vi "Pololu.Mgr - Connect.vi"(8 "error in (no error)":errorcluster, 9 "PID":string, 10 "VID":string, 11 "PololuCtrl in":refnum<class "PololuCtrl.lvclass">) -> (0 "error out":errorcluster, 2 "Com Port":refnum<visa-resource-name>, 3 "PololuCtrl out":refnum<class "PololuCtrl.lvclass">)   [LabVIEW 2018, in "PololuCtrl.lvclass"]
uses:
  PololuCtrl.lvclass
  Utils/Errors/Error.Error Code List.ctl
  PololuCtrl.lvclass/PololuCtrl.ctl
  Serial Port/Class/SerialPort.lvclass
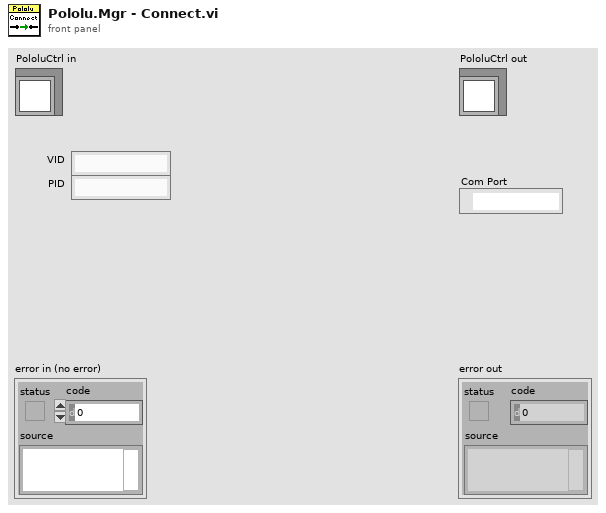
[diagram p1: front panel]
types:
  T1 = typedef "Error.Error Code List.ctl" = i32
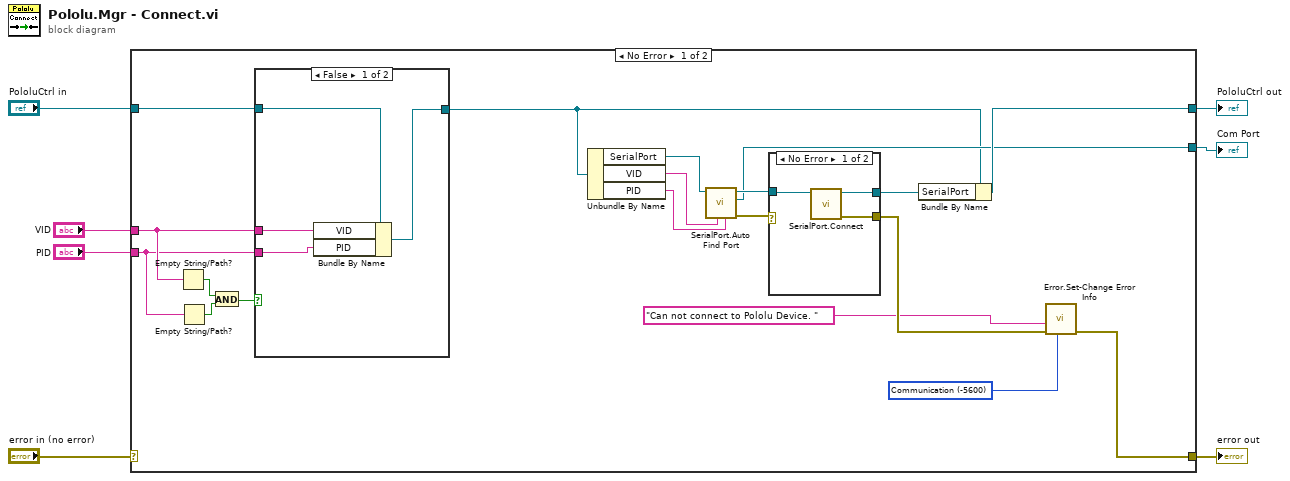
[diagram p0: block diagram]
diagram:
  n1 = case shown="No Error" "error in (no error)" {
    selector: "error in (no error)" -> [_ w38]
    tunnel: [w16 w38] -> w6
    tunnel: [w26 w37] -> w4
    tunnel: "PololuCtrl in" -> [w11 w37]
    tunnel: [w15 _] -> w3
    tunnel: "VID" -> [w9 _]
    tunnel: "PID" -> [w8 _]
    frame No Error {
      w18 = T1 -5600 items=["No Error"=0, "Abort"=-2, "Misc"=-5000, "Fixture Error"=-5100, "File IO - General"=-5200, "FIle IO - Config Error"=-5201, "Instrument - General"=-5300, "Instrument - Serial Com"=-5301, "Instrument - Camera"=-5302, "Instrument - PS"=-5303, "Instrument - Oscilloscope"=-5304, "Instrument - Function Gen"=-5305, "Instrument - Load"=-5306, "Instrument - Meter"=-5307, "Instrument - Power Control"=-5308, "Instrument - Motion"=-5309, "Instrument - RF"=-5310, "System Exe"=-5400, "Image Processing"=-5500, "Communication"=-5600, "Script - Syntax Error"=-6000, "Script - Invalid Name or Param"=-6100, "Script - Timeout"=-6200, "Invalid Data"=-6300, "FW Update Error"=-6500] ("Std Code")
      n2 = Empty String/Path?(string/path=w9) -> (empty?=w13:bool)
      n3 = Empty String/Path?(string/path=w8) -> (empty?=w14:bool)
      n4 = And(x=w13, y=w14) -> (x .and. y?=w12:bool)
      n5 = case shown="False" w12 {
        tunnel: w11 -> [w30 w31]
        tunnel: [w27 w31] -> w10
        tunnel: w9 -> [w29 _]
        tunnel: w8 -> [w28 _]
        frame False {
          n6 = Bundle By Name(cluster=w30, "VID"=w29, "PID"=w28) -> (w27:refnum<class "PololuCtrl.lvclass">)
        }
        frame True {
        }
      }
      n7 = Unbundle By Name(w10) -> ("SerialPort"=w25:refnum<class "SerialPort.lvclass">, "VID"=w24:string, "PID"=w23:string)
      n8 = call "SerialPort.Auto Find Port.vi"("PID"=w23, "VID"=w24, "SerialPort in"=w25) -> ("error out"=w22:errorcluster, "VISA resource name"=w15:refnum<visa-resource-name>, "SerialPort out"=w21:refnum<class "SerialPort.lvclass">)  [unwired: 6 in]
      n9 = case shown="No Error" w22 {
        selector: w22 -> [_ w36]
        tunnel: w21 -> [w34 w35]
        tunnel: [w33 w35] -> w20
        tunnel: [w32 w36] -> w19
        frame No Error {
          n10 = call "SerialPort.Connect.vi"("SerialPort in"=w34) -> ("error out"=w32:errorcluster, "SerialPort out"=w33:refnum<class "SerialPort.lvclass">)  [unwired: 8 in, 1 out]
        }
        frame Error {
        }
      }
      n11 = Bundle By Name(cluster=w10, "SerialPort"=w20) -> (w26:refnum<class "PololuCtrl.lvclass">)
      n12 = call "Error.Set-Change Error Info.vi"("Std Code"=w18, "error in"=w19, "Description"="Can not connect to Pololu Device. ") -> ("error out"=w16:errorcluster)  [unwired: 8 in]
    }
    frame Error {
    }
  }
  "error out" <- w6
  "PololuCtrl out" <- w4
  "Com Port" <- w3
